vi "configure gating.vi"(8 "error in (no error)":errorcluster, 9 "Board":u16, 10 "GatingMode":u32(ring) items=["FreeRunning", "TriggerRising", "TriggerFalling", "TriggerBoth", "GatedHigh", "GatedLow"], 11 "identifier":string) -> (0 "error out":errorcluster, 3 "function return":u32)   [LabVIEW 2015, in "XGL_DPP.lvlib"]
doc: "EXTERN DECLSPEC uint32_t CALL_CONV configure_gating(const char * identifier, const GatingMode GatingMode, uint16_t Board);"
uses:
  XGL_DPP.lvlib
  XGL_DPP.dll
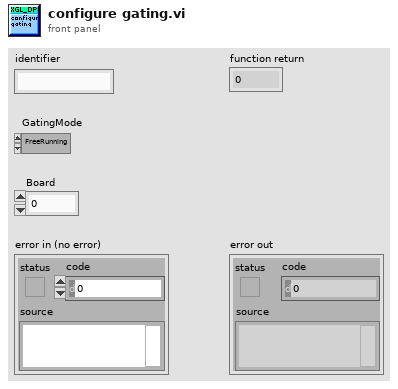
[diagram p1: front panel]
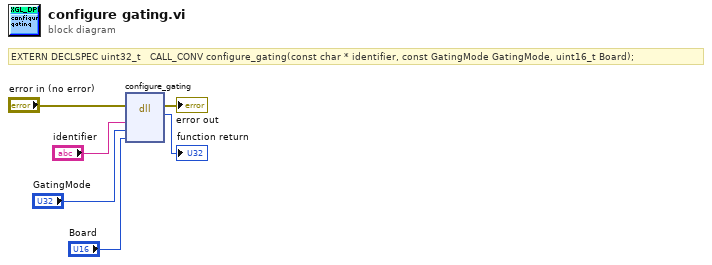
[diagram p0: block diagram]
diagram:
  # "EXTERN DECLSPEC uint32_t   CALL_CONV configure_gating(const char * identifier, const GatingMode GatingMode, uint16_t Board);"
  n1 = dll-call lib="D:/Users/XRF/Desktop/Scanning Software_Demokritos_2015_v7/libs/Vis_2/XGL_DPP.*" fn="configure_gating"(error in="error in (no error)", "identifier"="identifier", "GatingMode"="GatingMode", "Board"="Board") -> (error out=→"error out":errorcluster, →"function return":u32)  [unwired: 5 in, 1 out]
